vi "Find Missing.vi"(6 "Maze (0: Empty, -1: Enemy. >0: Teammate":i32[][](array[numeric]), 7 "known_p in":i32, 9 "Move":i32, 10 "Assumed Board":i32[][](array[numeric]), 11 "Info[p]":T1[](array[typedef])) -> (1 "Found?":bool, 3 "Info[p] out":T1[](array[typedef]), 5 "known_p out":i32)   [LabVIEW 2015, in "TeamEffort.lvclass"]
uses:
  TeamEffort.lvclass
  private/Player Cluster.ctl
  Square/Square.lvclass
  Team Move Input.ctl
  Type Defs/Action Enum.ctl
  Team Move Output.ctl
  Type Defs/Direction Enum.ctl
  Type Defs/SB Type Defs.lvlib
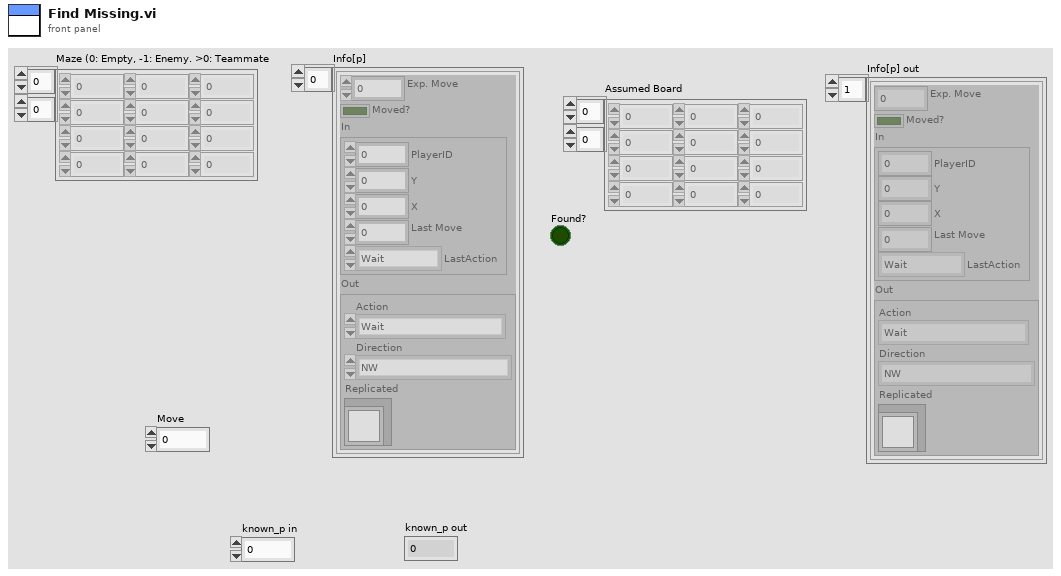
[diagram p1: front panel]
types:
  T1 = typedef "TeamEffort.lvclass/Player Cluster.ctl" = cluster{"Exp. Move":i32, "Moved?":bool, "In":T2, "Out":T4}
  T2 = typedef "TeamEffort.lvclass/Team Move Input.ctl" = cluster{"PlayerID":i32, "Y":i32, "X":i32, "Last Move":i32, "LastAction":T3}
  T3 = typedef "SB Type Defs.lvlib/Action Enum.ctl" = enum16{"Wait", "Move", "Attack", "Replicate"}
  T4 = typedef "TeamEffort.lvclass/Team Move Output.ctl" = cluster{"Action":T3, "Direction":T5, "Replicated":refnum<class "Square.lvclass">}
  T5 = typedef "SB Type Defs.lvlib/Direction Enum.ctl" = enum16{"NW", "N", "NE", "E", "SE", "S", "SW", "W"}
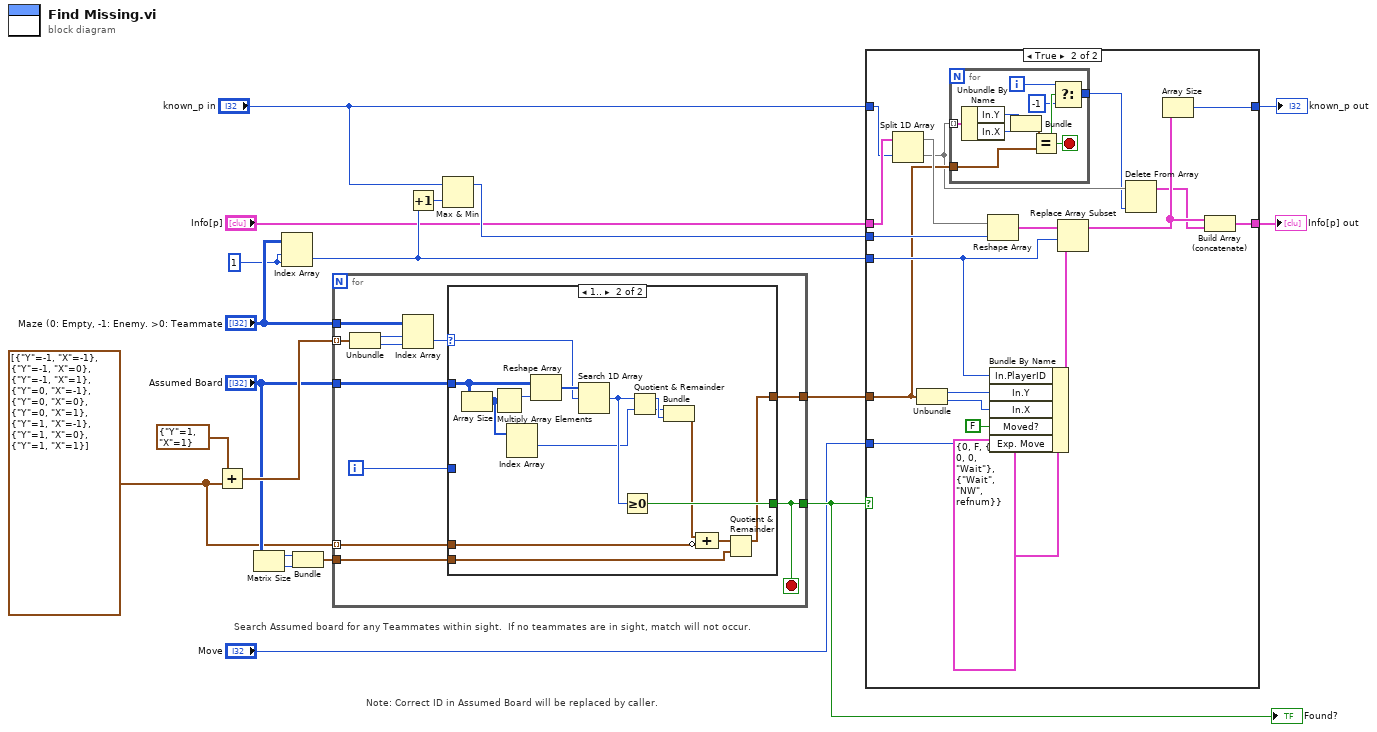
[diagram p0: block diagram]
diagram:
  w18 = 1 ("disabled index (col)")
  w4 = cluster{"Y":i32, "X":i32}[] [{"Y"=-1, "X"=-1}, {"Y"=-1, "X"=0}, {"Y"=-1, "X"=1}, {"Y"=0, "X"=-1}, {"Y"=0, "X"=0}, {"Y"=0, "X"=1}, {"Y"=1, "X"=-1}, {"Y"=1, "X"=0}, {"Y"=1, "X"=1}]
  # "Search Assumed board for any Teammates within sight.  If no teammates are in sight, match will not occur."
  # "Note: Correct ID in Assumed Board will be replaced by caller."
  n1 = Add(x=cluster{"Y":i32, "X":i32} {"Y"=1, "X"=1}, y=w4) -> (x+y=w9:cluster{"Y":i32, "X":i32}[])
  n2 = Matrix Size(0:"Assumed Board") -> (1:w7:i32, 2:w6:i32)
  n3 = Index Array(array="Maze (0: Empty, -1: Enemy. >0: Teammate", index (row)=w18, index (col)=w18) -> (element=w12:i32)
  n4 = Bundle("number of columns"=w7, "matrix"=w6) -> (w5:cluster{"number of columns":i32, "matrix":i32})  [unwired: 1 in]
  n5 = for {
    tunnel: "Maze (0: Empty, -1: Enemy. >0: Teammate" -> [w30]
    tunnel: w9 -> [w22] mode=indexing
    tunnel: "Assumed Board" -> [w26]
    tunnel: [w25] -> w13
    tunnel: [w24] -> w14
    tunnel: w5 -> [w21]
    tunnel: w4 -> [w20] mode=indexing
    i -> [w23]
    stop <- w24 stop-if-true
    n6 = Unbundle(w22) -> ("Y"=w29:i32, "X"=w28:i32)
    n7 = Index Array(array=w30, index (row)=w29, index (col)=w28) -> (element=w27:i32)
    n8 = case shown="1.." w27 {
      selector: w27 -> [_ w42]
      tunnel: w26 -> [_ w45]
      tunnel: [_ w41] -> w24
      tunnel: [_ w31] -> w25
      tunnel: w23 -> [_ _]
      tunnel: w20 -> [_ w37]
      tunnel: w21 -> [_ w32]
      frame ..0 {
      }
      frame 1.. {
        n9 = Array Size(array=w45) -> (size(s)=w39:i32[])
        n10 = Multiply Array Elements(1:w39) -> (0:w44:i32)
        n11 = Index Array(array=w39) -> (element #1=w38:i32)  [unwired: 2 in, 1 out]
        n12 = Reshape Array(w45, w44) -> (w43:i32[])
        n13 = Search 1D Array(1D array=w43, element=w42) -> (index of element=w40:i32)  [unwired: 1 in]
        n14 = Greater Or Equal To 0?(x=w40) -> (x >= 0?=w41:bool)
        n15 = Quotient & Remainder(x=w40, y=w38) -> (x-y*floor(x/y)=w36:i32, floor(x/y)=w35:i32)
        n16 = Bundle(w35, w36) -> (w34:cluster{i32, i32})  [unwired: 1 in]
        n17 = Compound Arithmetic op=ADD(w34, invert w37) -> (w33:cluster{i32, i32})
        n18 = Quotient & Remainder(x=w33, y=w32) -> (x-y*floor(x/y)=w31:cluster{i32, i32})  [unwired: 1 out]
      }
    }
  }
  "Found?" <- w14
  n19 = Increment(x=w12) -> (x+1=w17:i32)
  n20 = Max & Min(x="known_p in", y=w17) -> (max(x,y)=w16:i32)  [unwired: 1 out]
  n21 = case shown="True" w14 {
    tunnel: "Info[p]" -> [w47 w59]
    tunnel: w16 -> [_ w66]
    tunnel: [w47 w55] -> w15
    tunnel: w13 -> [_ w52]
    tunnel: w12 -> [_ w64]
    tunnel: "Move" -> [_ w61]
    tunnel: "known_p in" -> [w46 w58]
    tunnel: [w46 w53] -> w3
    frame False {
    }
    frame True {
      n22 = Split 1D Array(array=w59, index=w58) -> (first subarray=w57:T1[], second subarray=w51:T1[])
      n23 = Unbundle(w52) -> (w48:i32, w60:i32)
      n24 = for {
        tunnel: w51 -> [w75] mode=indexing
        tunnel: w52 -> [w72]
        tunnel: [w67] -> w50
        i -> [w69]
        stop <- w70 stop-if-true
        n25 = Unbundle By Name(w75) -> ("In.Y"=w74:i32, "In.X"=w73:i32)
        n26 = Bundle("Y"=w74, "X"=w73) -> (w71:cluster{"Y":i32, "X":i32})  [unwired: 1 in]
        n27 = Equal?(x=w71, y=w72) -> (x = y?=w70:bool)
        n28 = Select(t=w69, s=w70, f=-1) -> (s? t:f=w67:i32)
      }
      n29 = Reshape Array(w57, w66) -> (w56:T1[])
      n30 = Bundle By Name(cluster=T1 {"Exp. Move"=0, "Moved?"=FALSE, "In"={"PlayerID"=0, "Y"=0, "X"=0, "Last Move"=0, "LastAction"=enum."Wait"}, "Out"={"Action"=enum."Wait", "Direction"=enum."NW", "Replicated"=refnum}} ("new element/subarray"), "In.PlayerID"=w64, "In.Y"=w48, "In.X"=w60, "Moved?"=FALSE, "Exp. Move"=w61) -> (w62:T1)
      n31 = Replace Array Subset(array=w56, new element=w62, index=w64) -> (w54:T1[])
      n32 = Delete From Array(array=w51, index=w50) -> (array with subset deleted=w49:T1[])  [unwired: 1 in, 1 out]
      n33 = Array Size(array=w54) -> (size(s)=w53:i32)
      n34 = Build Array (concatenate)(w54, w49) -> (w55:T1[])
    }
  }
  "Info[p] out" <- w15
  "known_p out" <- w3
